vi "Untitled 5.vi"() -> ()   [LabVIEW 2013]
uses:
  Parsing State.ctl
  JSONtext.lvlib
panel:
  out "Array":cluster{T1, bool}[](array[cluster])
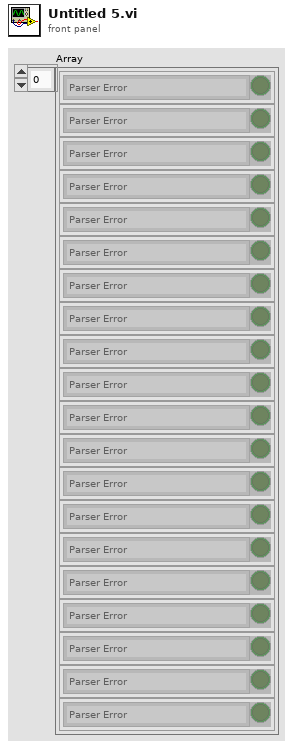
[diagram p1: front panel]
types:
  T1 = typedef "JSONtext.lvlib/Parsing State.ctl" = enum16{"Parser Error", "Object", "Array", "String", "Number/Other", "Leading Whitespace", "Object end", "Array end", "Value end"}
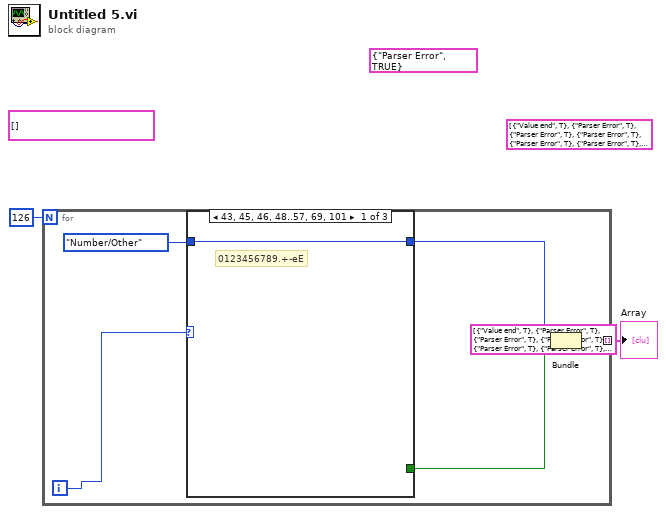
[diagram p0: block diagram]
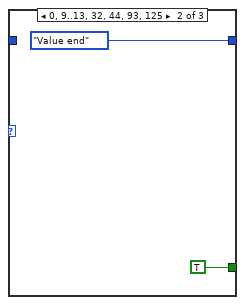
[diagram p2: hidden frame]
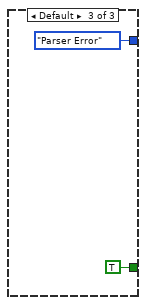
[diagram p3: hidden frame]
diagram:
  (unwired) cluster{T1, bool}[] [{enum."Value end", TRUE}, {enum."Parser Error", TRUE}, {enum."Parser Error", TRUE}, {enum."Parser Error", TRUE}, {enum."Parser Error", TRUE}, {enum."Parser Error", TRUE}, {enum."Parser Error", TRUE}, {enum."Parser Error", TRUE}, {enum."Parser Error", TRUE}, {enum."Value end", TRUE}, {enum."Value end", TRUE}, {enum."Value end", TRUE}, {enum."Value end", TRUE}, {enum."Value end", TRUE}, {enum."Parser Error", TRUE}, {enum."Parser Error", TRUE}, {enum."Parser Error", TRUE}, {enum."Parser Error", TRUE}, {enum."Parser Error", TRUE}, {enum."Parser Error", TRUE}, {enum."Parser Error", TRUE}, {enum."Parser Error", TRUE}, {enum."Parser Error", TRUE}, {enum."Parser Error", TRUE}, {enum."Parser Error", TRUE}, {enum."Parser Error", TRUE}, {enum."Parser Error", TRUE}, {enum."Parser Error", TRUE}, {enum."Parser Error", TRUE}, {enum."Parser Error", TRUE}, {enum."Parser Error", TRUE}, {enum."Parser Error", TRUE}, {enum."Value end", TRUE}, {enum."Parser Error", TRUE}, {enum."Parser Error", TRUE}, {enum."Parser Error", TRUE}, {enum."Parser Error", TRUE}, {enum."Parser Error", TRUE}, {enum."Parser Error", TRUE}, {enum."Parser Error", TRUE}, {enum."Parser Error", TRUE}, {enum."Parser Error", TRUE}, {enum."Parser Error", TRUE}, {enum."Number/Other", FALSE}, {enum."Value end", TRUE}, {enum."Number/Other", FALSE}, {enum."Number/Other", FALSE}, {enum."Parser Error", TRUE}, {enum."Number/Other", FALSE}, {enum."Number/Other", FALSE}, {enum."Number/Other", FALSE}, {enum."Number/Other", FALSE}, {enum."Number/Other", FALSE}, {enum."Number/Other", FALSE}, {enum."Number/Other", FALSE}, {enum."Number/Other", FALSE}, {enum."Number/Other", FALSE}, {enum."Number/Other", FALSE}, {enum."Parser Error", TRUE}, {enum."Parser Error", TRUE}, {enum."Parser Error", TRUE}, {enum."Parser Error", TRUE}, {enum."Parser Error", TRUE}, {enum."Parser Error", TRUE}, {enum."Parser Error", TRUE}, {enum."Parser Error", TRUE}, {enum."Parser Error", TRUE}, {enum."Parser Error", TRUE}, {enum."Parser Error", TRUE}, {enum."Number/Other", FALSE}, {enum."Parser Error", TRUE}, {enum."Parser Error", TRUE}, {enum."Parser Error", TRUE}, {enum."Parser Error", TRUE}, {enum."Parser Error", TRUE}, {enum."Parser Error", TRUE}, {enum."Parser Error", TRUE}, {enum."Parser Error", TRUE}, {enum."Parser Error", TRUE}, {enum."Parser Error", TRUE}, {enum."Parser Error", TRUE}, {enum."Parser Error", TRUE}, {enum."Parser Error", TRUE}, {enum."Parser Error", TRUE}, {enum."Parser Error", TRUE}, {enum."Parser Error", TRUE}, {enum."Parser Error", TRUE}, {enum."Parser Error", TRUE}, {enum."Parser Error", TRUE}, {enum."Parser Error", TRUE}, {enum."Parser Error", TRUE}, {enum."Parser Error", TRUE}, {enum."Parser Error", TRUE}, {enum."Value end", TRUE}, {enum."Parser Error", TRUE}, {enum."Parser Error", TRUE}, {enum."Parser Error", TRUE}, {enum."Parser Error", TRUE}, {enum."Parser Error", TRUE}, {enum."Parser Error", TRUE}, {enum."Parser Error", TRUE}, {enum."Number/Other", FALSE}, {enum."Parser Error", TRUE}, {enum."Parser Error", TRUE}, {enum."Parser Error", TRUE}, {enum."Parser Error", TRUE}, {enum."Parser Error", TRUE}, {enum."Parser Error", TRUE}, {enum."Parser Error", TRUE}, {enum."Parser Error", TRUE}, {enum."Parser Error", TRUE}, {enum."Parser Error", TRUE}, {enum."Parser Error", TRUE}, {enum."Parser Error", TRUE}, {enum."Parser Error", TRUE}, {enum."Parser Error", TRUE}, {enum."Parser Error", TRUE}, {enum."Parser Error", TRUE}, {enum."Parser Error", TRUE}, {enum."Parser Error", TRUE}, {enum."Parser Error", TRUE}, {enum."Parser Error", TRUE}, {enum."Parser Error", TRUE}, {enum."Parser Error", TRUE}, {enum."Parser Error", TRUE}, {enum."Value end", TRUE}] ("Array")
  (unwired) cluster{T1, bool}[] [{enum."Value end", TRUE}, {enum."Parser Error", TRUE}, {enum."Parser Error", TRUE}, {enum."Parser Error", TRUE}, {enum."Parser Error", TRUE}, {enum."Parser Error", TRUE}, {enum."Parser Error", TRUE}, {enum."Parser Error", TRUE}, {enum."Parser Error", TRUE}, {enum."Value end", TRUE}, {enum."Value end", TRUE}, {enum."Value end", TRUE}, {enum."Value end", TRUE}, {enum."Value end", TRUE}, {enum."Parser Error", TRUE}, {enum."Parser Error", TRUE}, {enum."Parser Error", TRUE}, {enum."Parser Error", TRUE}, {enum."Parser Error", TRUE}, {enum."Parser Error", TRUE}, {enum."Parser Error", TRUE}, {enum."Parser Error", TRUE}, {enum."Parser Error", TRUE}, {enum."Parser Error", TRUE}, {enum."Parser Error", TRUE}, {enum."Parser Error", TRUE}, {enum."Parser Error", TRUE}, {enum."Parser Error", TRUE}, {enum."Parser Error", TRUE}, {enum."Parser Error", TRUE}, {enum."Parser Error", TRUE}, {enum."Parser Error", TRUE}, {enum."Value end", TRUE}, {enum."Parser Error", TRUE}, {enum."Parser Error", TRUE}, {enum."Parser Error", TRUE}, {enum."Parser Error", TRUE}, {enum."Parser Error", TRUE}, {enum."Parser Error", TRUE}, {enum."Parser Error", TRUE}, {enum."Parser Error", TRUE}, {enum."Parser Error", TRUE}, {enum."Parser Error", TRUE}, {enum."Number/Other", FALSE}, {enum."Value end", TRUE}, {enum."Number/Other", FALSE}, {enum."Number/Other", FALSE}, {enum."Parser Error", TRUE}, {enum."Number/Other", FALSE}, {enum."Number/Other", FALSE}, {enum."Number/Other", FALSE}, {enum."Number/Other", FALSE}, {enum."Number/Other", FALSE}, {enum."Number/Other", FALSE}, {enum."Number/Other", FALSE}, {enum."Number/Other", FALSE}, {enum."Number/Other", FALSE}, {enum."Number/Other", FALSE}, {enum."Parser Error", TRUE}, {enum."Parser Error", TRUE}, {enum."Parser Error", TRUE}, {enum."Parser Error", TRUE}, {enum."Parser Error", TRUE}, {enum."Parser Error", TRUE}, {enum."Parser Error", TRUE}, {enum."Parser Error", TRUE}, {enum."Parser Error", TRUE}, {enum."Parser Error", TRUE}, {enum."Parser Error", TRUE}, {enum."Number/Other", FALSE}, {enum."Parser Error", TRUE}, {enum."Parser Error", TRUE}, {enum."Parser Error", TRUE}, {enum."Parser Error", TRUE}, {enum."Parser Error", TRUE}, {enum."Parser Error", TRUE}, {enum."Parser Error", TRUE}, {enum."Parser Error", TRUE}, {enum."Parser Error", TRUE}, {enum."Parser Error", TRUE}, {enum."Parser Error", TRUE}, {enum."Parser Error", TRUE}, {enum."Parser Error", TRUE}, {enum."Parser Error", TRUE}, {enum."Parser Error", TRUE}, {enum."Parser Error", TRUE}, {enum."Parser Error", TRUE}, {enum."Parser Error", TRUE}, {enum."Parser Error", TRUE}, {enum."Parser Error", TRUE}, {enum."Parser Error", TRUE}, {enum."Parser Error", TRUE}, {enum."Parser Error", TRUE}, {enum."Value end", TRUE}, {enum."Parser Error", TRUE}, {enum."Parser Error", TRUE}, {enum."Parser Error", TRUE}, {enum."Parser Error", TRUE}, {enum."Parser Error", TRUE}, {enum."Parser Error", TRUE}, {enum."Parser Error", TRUE}, {enum."Number/Other", FALSE}, {enum."Parser Error", TRUE}, {enum."Parser Error", TRUE}, {enum."Parser Error", TRUE}, {enum."Parser Error", TRUE}, {enum."Parser Error", TRUE}, {enum."Parser Error", TRUE}, {enum."Parser Error", TRUE}, {enum."Parser Error", TRUE}, {enum."Parser Error", TRUE}, {enum."Parser Error", TRUE}, {enum."Parser Error", TRUE}, {enum."Parser Error", TRUE}, {enum."Parser Error", TRUE}, {enum."Parser Error", TRUE}, {enum."Parser Error", TRUE}, {enum."Parser Error", TRUE}, {enum."Parser Error", TRUE}, {enum."Parser Error", TRUE}, {enum."Parser Error", TRUE}, {enum."Parser Error", TRUE}, {enum."Parser Error", TRUE}, {enum."Parser Error", TRUE}, {enum."Parser Error", TRUE}] ("Array")
  (unwired) cluster{T1, bool} {enum."Parser Error", TRUE}
  (unwired) cluster{T1, bool}[] []
  n1 = for {
    N: 126 -> [_]
    tunnel: [w3] -> w1 mode=indexing
    i -> [w7]
    n2 = case shown="43, 45, 46, 48..57, 69, 101" w7 {
      tunnel: Parsing_State."Number/Other" -> [w8 _ _]
      tunnel: [w8 Parsing_State."Value end" Parsing_State."Parser Error"] -> w5
      tunnel: [_ TRUE TRUE] -> w4
      frame 43, 45, 46, 48..57, 69, 101 {
        # "0123456789.+-eE"
      }
      frame 0, 9..13, 32, 44, 93, 125 {
      }
      frame Default {
      }
    }
    n3 = Bundle(w5, w4) -> (w3:cluster{T1, bool})  [unwired: 1 in]
  }
  "Array" <- w1
